vi "Read 3D Pie Property Array.vi"(8 "error in (no error)":errorcluster, 11 "3D Pie.lvclass in":refnum<class "3D Pie.lvclass">) -> (0 "error out":errorcluster, 2 "3D Pie Property Array":T1, 3 "3D Pie.lvclass out":refnum<class "3D Pie.lvclass">)   [LabVIEW 2017, in "3D Pie.lvclass"]
uses:
  <vilib>/Math Plots/3D Math Plots/3D Pie/3D Pie/3D Pie.lvclass
  <vilib>/Math Plots/3D Math Plots/3D Pie/3D Pie/Typedef/3D Pie Property Array.ctl
  <vilib>/Math Plots/3D Math Plots/3D Pie/3D Pie/Typedef/3D Pie Property.ctl
  <vilib>/Math Plots/3D Math Plots/3D Plot/3D Plot/Typedef/Line Type.ctl
  <vilib>/Math Plots/3D Math Plots/3D Pie/3D Pie/3D Pie.lvclass/3D Pie.ctl
  <vilib>/Math Plots/3D Math Plots/3D Plot/3D Plot/3D Plot.lvclass
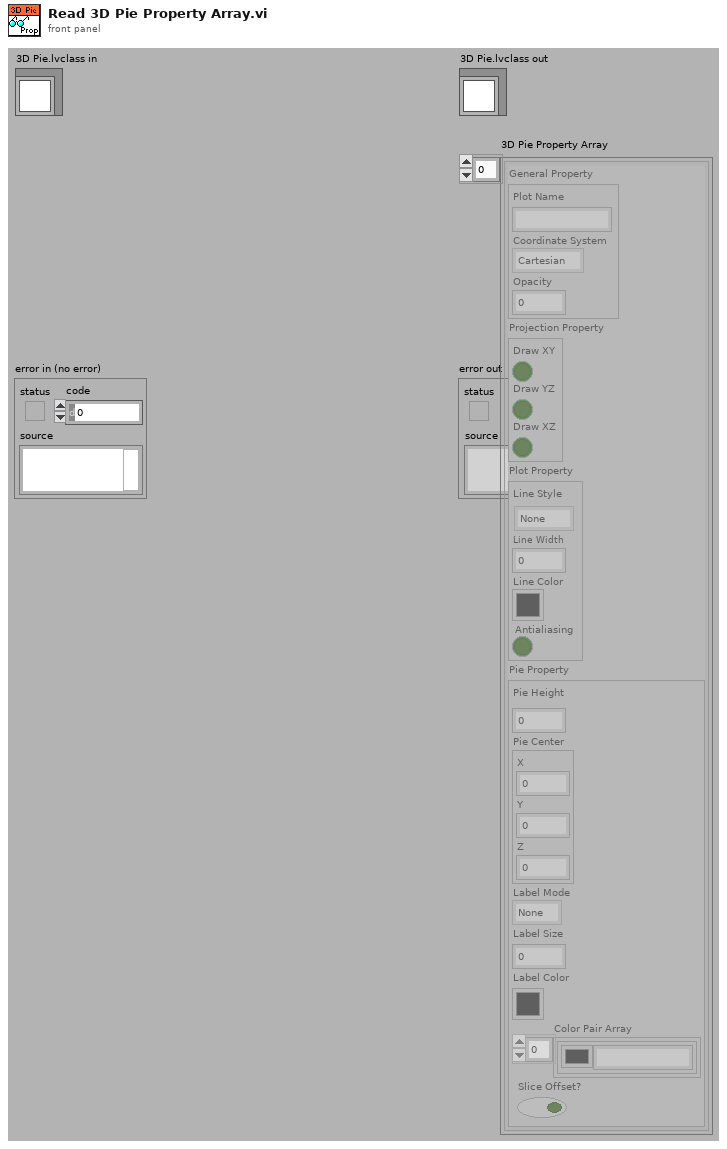
[diagram p1: front panel]
types:
  T1 = typedef "3D Pie.lvclass/3D Pie Property Array.ctl" = T2[]
  T2 = typedef "3D Pie.lvclass/3D Pie Property.ctl" = cluster{"General Property":cluster{"Plot Name":string, "Coordinate System":enum16{"Cartesian", "Cylindrical", "Spherical"}, "Opacity":sgl}, "Projection Property":cluster{"Draw XY":bool, "Draw YZ":bool, "Draw XZ":bool}, "Plot Property":cluster{"Line Style":T3, "Line Width":sgl, "Line Color":u32, "Antialiasing":bool}, "Pie Property":cluster{"Pie Height":sgl, "Pie Center":cluster{"X":sgl, "Y":sgl, "Z":sgl}, "Label Mode":enum16{"None", "Show Percentage", "Show String"}, "Label Size":u16, "Label Color":u32, "Color Pair Array":cluster{"Color":u32, "String":string}[], "Slice Offset?":bool}}
  T3 = typedef "3D Plot.lvclass/Line Type.ctl" = enum16{"None", "Solid", "Dash", "Dot", "Dash Dot"}
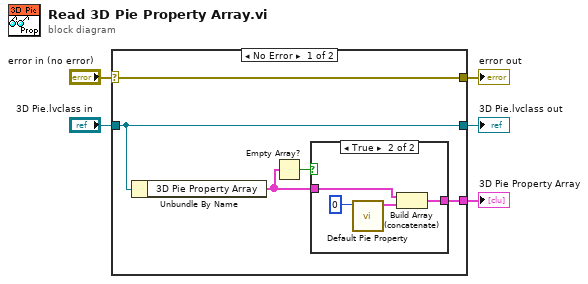
[diagram p0: block diagram]
diagram:
  n1 = case shown="No Error" "error in (no error)" {
    selector: "error in (no error)" -> [w10 w16]
    tunnel: [w10 w16] -> w4
    tunnel: [w9 w17] -> w2
    tunnel: "3D Pie.lvclass in" -> [w9 w17]
    tunnel: [w6 _] -> w1
    frame No Error {
      n2 = Unbundle By Name(w9) -> ("3D Pie Property Array"=w7:T1)
      n3 = Empty Array?(array=w7) -> (empty?=w8:bool)
      n4 = case shown="True" w8 {
        tunnel: w7 -> [w11 w14]
        tunnel: [w11 w13] -> w6
        frame False {
        }
        frame True {
          n5 = call <vilib>:"Default Pie Property.vi"("Plot ID"=0) -> ("Default Property"=w15:T2)  [unwired: 10 in]
          n6 = Build Array (concatenate)(w14, w15) -> (w13:T1)
        }
      }
    }
    frame Error {
    }
  }
  "error out" <- w4
  "3D Pie.lvclass out" <- w2
  "3D Pie Property Array" <- w1
